vi "Ocean Optics Driver.vi"() -> ()   [LabVIEW 2023]
uses:
  <vilib>/event_ctls.llb/lveventtype.ctl
  <vilib>/Utility/inputDevices.llb/mouseAcquire.vi
  <vilib>/express/express shared/transition.llb/Dynamic To Waveform Array.vi
  <vilib>/express/express signal manip/GetorSetDDTAttributes/Set DDT Attributes/SetT0.vi
  <vilib>/express/express shared/transition.llb/Waveform Array To Dynamic.vi
  <vilib>/express/express signal manip/GetorSetDDTAttributes/Set DDT Attributes/Set DDT Properties.xnode
panel:
  in  "Excitation power:":dbl=84.0 format="%d mW"
  out "Saving Data":bool
  in  "save":bool
  in  "Subtract bckg.":bool
  in  "Background":bool
  in  "length":i32=2 min=0 max=100 step=1
  in  "History mode":bool
  in  "Enable cal":bool
  in  "Calibration consants:":dbl[](array[numeric])=[-1.0164322463e-05, 1.0203031499, -10.120763965] format="%#_6e"
  in  "Raman ref:":dbl=532.0 format="%#_g nm"
  in  "Units":bool=TRUE
  out "Cursor Position:":dbl
  out "XY Graph":cluster{dbl[], "Spectrum Values":dbl[]}[](graph)
  in  "Integration time:":dbl=0.1 min=0.001 max=60.0 step=0.01 format="%#_f s"
  out "Serial Number:":string
  in  "Media Stop Button":bool
  in  "Play":bool
  in  "EXIT":bool
  out "Data":cluster{dbl[], "Spectrum Values":dbl[]}[](array[cluster])
  out "Background":dbl[](array[numeric])
  out "History mode data":cluster{dbl[], "Spectrum Values":dbl[]}[](array[cluster])
  # "2nd:"
  # "1st:"
  # "cm-1"
  # "nm"
  # "0th:"
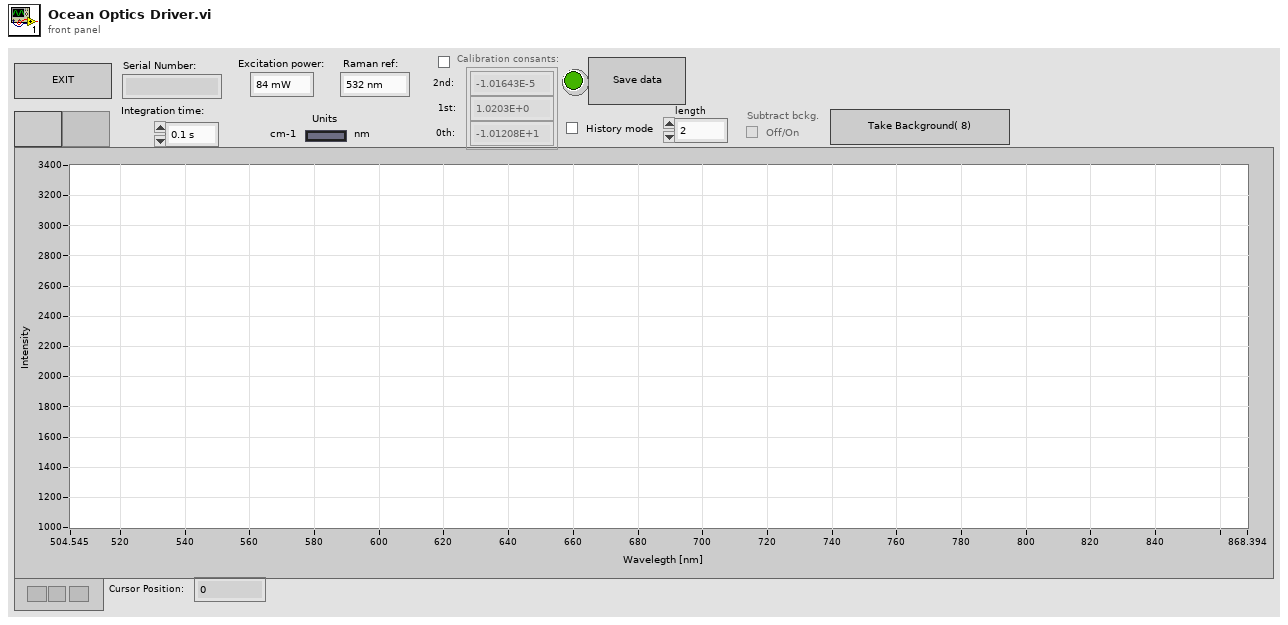
[diagram p1: front panel]
types:
  T1 = enum8{"Enabled", "Disabled", "Disabled and Grayed Out"}
  T2 = typedef "lveventtype.ctl" = enum32{"Null", "Timeout", "Annotation Menu Selection", "Annotation Menu Selection?", "App Instance Close", "App Instance Close?", "Autoscale Range Change", "Bookmark Info Change", "Cell Edit", "Cell Edit?", "Cursor Grab", "Cursor Grab?", "Cursor Menu Selection", "Cursor Menu Selection?", "Cursor Move", "Cursor Release", "Data Change", "Direction Change", "Display State Change", "Drag Ended", "Drag Enter", "Drag Leave", "Drag Over", "Drag Source Update", "Drag Starting", "Drag Starting?", "Drop", "Exec State Change", "Key Down", "Key Down?", "Key Repeat", "Key Repeat?", "Key Up", "Listbox Double Click", "Menu Activation?", "Menu Selection (App)", "Menu Selection? (App)", "Menu Selection (User)", "Mouse Down", "Mouse Down?", "Mouse Enter", "Mouse Leave", "Mouse Move", "Mouse Up", "Mouse Wheel", "NI Security User Change (App)", "Pane Size", "Panel Close", "Panel Close?", "Panel Resize", "Plot Attribute Change", "Scale Range Change", "Shortcut Menu Activation?", "Shortcut Menu Selection (App)", "Shortcut Menu Selection? (App)", "Shortcut Menu Selection (User)", "Tree Double Click", "Tree Drag", "Tree Drag?", "Tree Drop", "Tree Drop?", "Tree Item Close", "Tree Item Close?", "Tree Item Open", "Tree Item Open?", "User Event", "Value Change"}
  T3 = cluster{"Horizontal":i32, "Vertical":i32, "Scrolling":i32}
  T4 = cluster{"button 1":bool, "button 2":bool, "button 3":bool, "button 4":bool}
  T5 = typedef "LVRectTypeDef.ctl" = cluster{"Left":i16, "Top":i16, "Right":i16, "Bottom":i16}
  T6 = cluster{"XScale.Maximum":dbl, "YScale.Maximum":dbl}
  T7 = cluster{"XScale.Minimum":dbl, "YScale.Minimum":dbl}
  T8 = cluster{"event type or object":T2, "event type or object":T2}
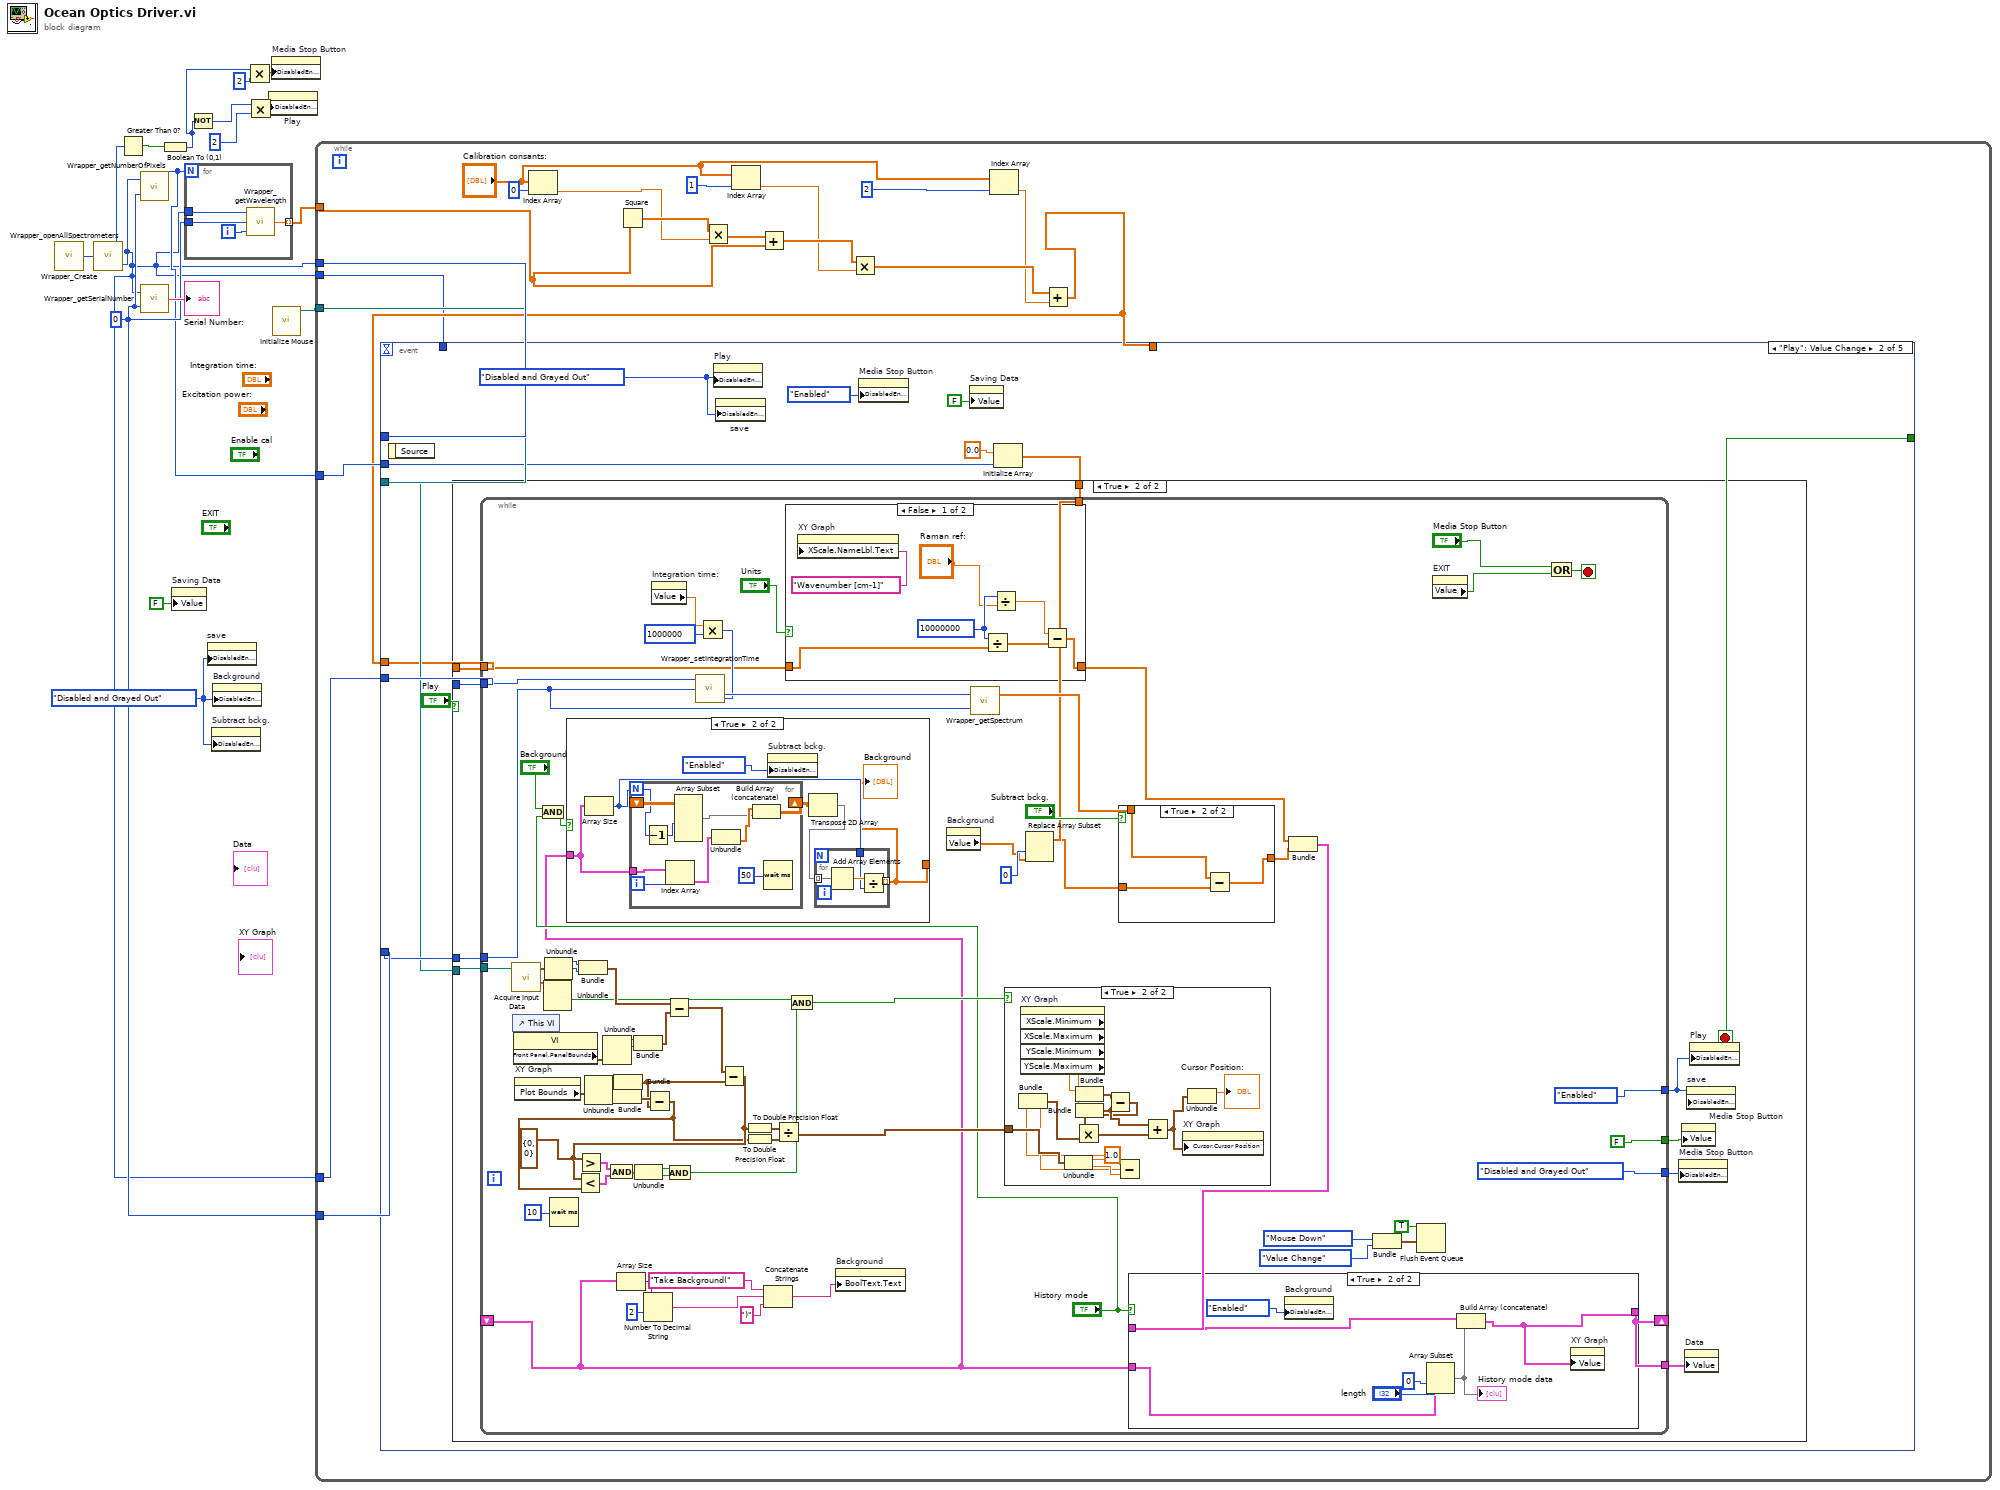
[diagram p0: block diagram]
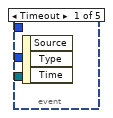
[diagram p2: hidden frame]
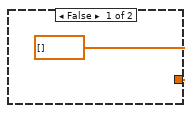
[diagram p5: hidden frame]
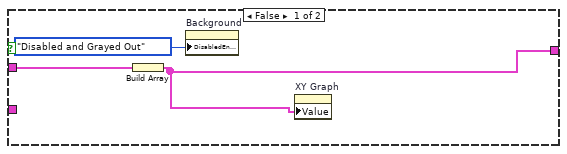
[diagram p6: hidden frame]
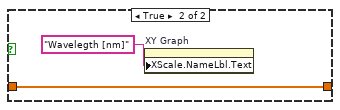
[diagram p7: hidden frame]
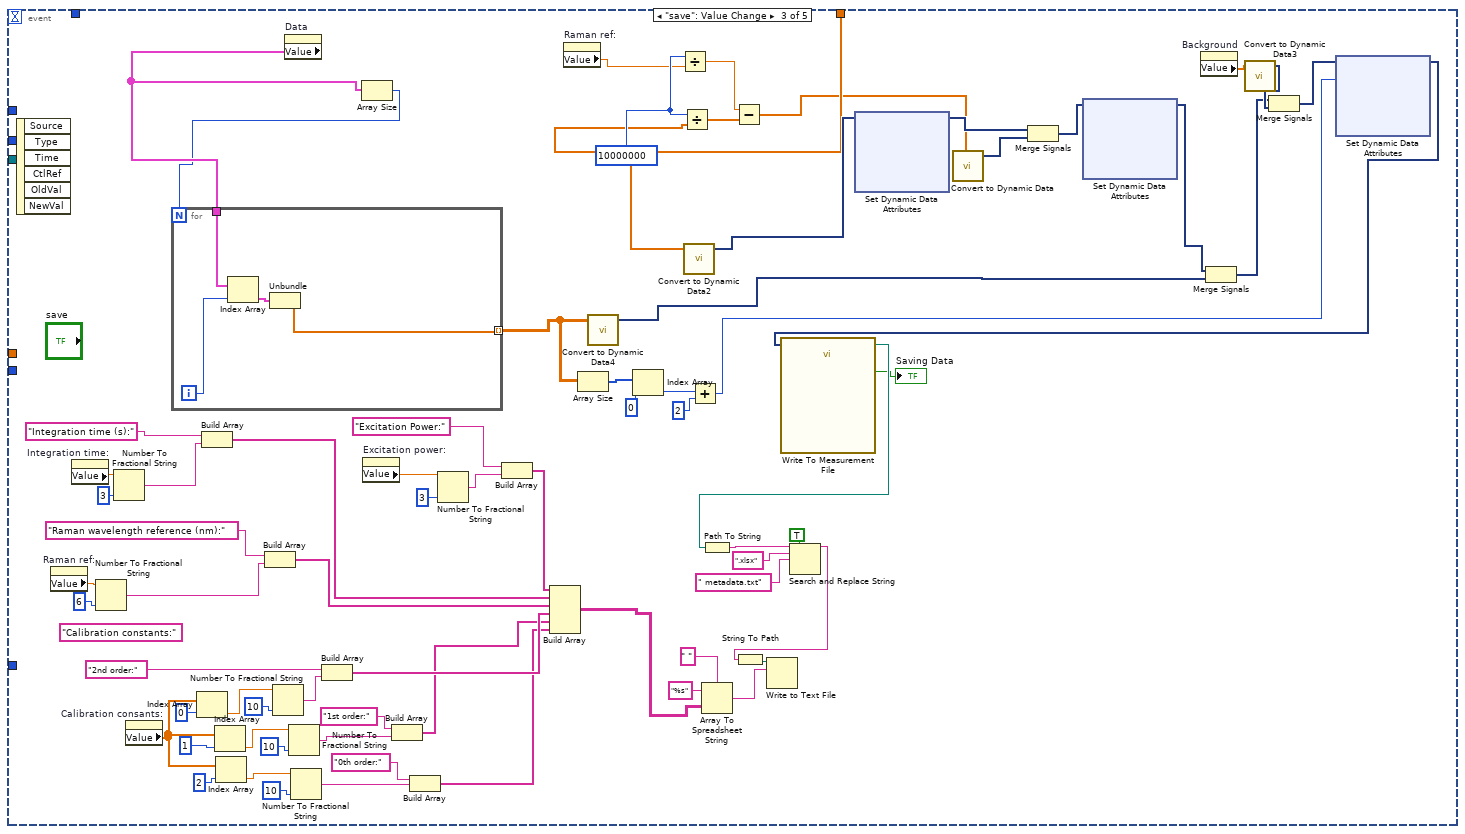
[diagram p9: hidden frame]
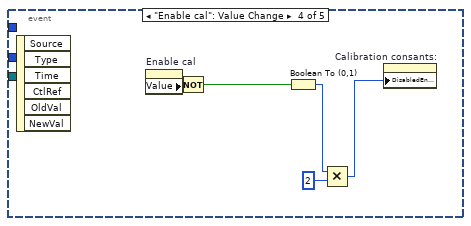
[diagram p10: hidden frame]
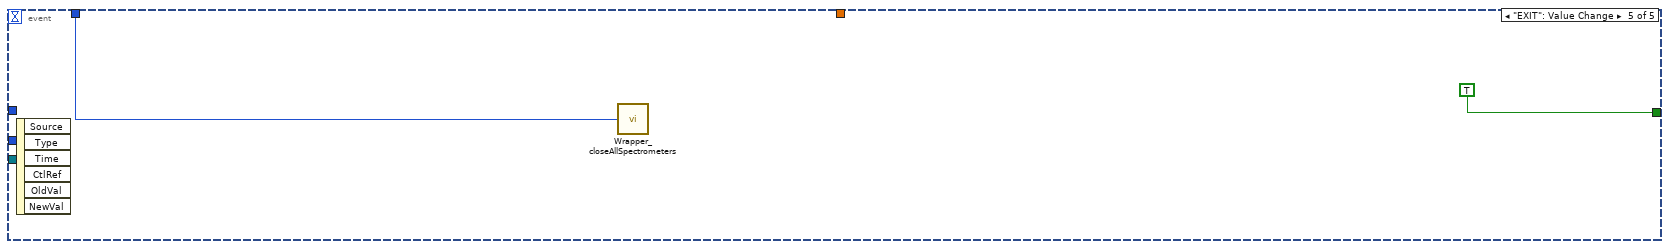
[diagram p11: hidden frame]
diagram:
  w2 = T1."Disabled and Grayed Out" ("Disabled")
  w15 = 0
  n1 = call "Wrapper_Create.vi"() -> ("Wrapper"=w17:u64)
  n2 = call "Wrapper_openAllSpectrometers.vi"("Wrapper In"=w17) -> ("Number of Spectrometers"=w13:i32, "Wrapper Out"=w1:u64)
  n3 = Greater Than 0?(x=w13) -> (x > 0?=w12:bool)
  n4 = call "Wrapper_getNumberOfPixels.vi"("Index"=w15, "Wrapper"=w1) -> ("Number of Pixels"=w4:i32)
  n5 = call "Wrapper_getSerialNumber.vi"("Index"=w15, "Wrapper"=w1) -> ("Serial Number"=→"Serial Number:":string)
  n6 = Boolean To (0,1)(Boolean=w12) -> (0, 1=w6:i16)
  n7 = property on="Saving Data" class="Bool (strict)"("Value"=FALSE ("Saving Data")) -> ()  [unwired: 2 in, 2 out]
  n8 = for {
    N: w4 -> [_]
    tunnel: w1 -> [w21]
    tunnel: w15 -> [w20]
    tunnel: [w18] -> w14 mode=indexing
    i -> [w19]
    n9 = call "Wrapper_getWavelength.vi"("Pixel"=w19, "Spectrometer Index"=w20, "Wrapper"=w21) -> ("Wavelength"=w18:dbl)
  }
  n10 = Not(x=w6) -> (.not. x?=w10:i16)
  n11 = property on="save" class="Bool"("DisabledEnum"=w2) -> ()  [unwired: 2 in, 2 out]
  n12 = property on="Subtract bckg." class="Bool (strict)"("DisabledEnum"=w2) -> ()  [unwired: 2 in, 2 out]
  n13 = property on="Background" class="Bool"("DisabledEnum"=w2) -> ()  [unwired: 2 in, 2 out]
  n14 = Multiply(x=w6, y=2) -> (x*y=w5:i32)
  n15 = Multiply(x=w10, y=2) -> (x*y=w9:i32)
  n16 = property on="Play" class="Bool"("DisabledEnum"=w9) -> ()  [unwired: 2 in, 2 out]
  n17 = property on="Media Stop Button" class="Bool (strict)"("DisabledEnum"=w5) -> ()  [unwired: 2 in, 2 out]
  n18 = call <vilib>:"Initialize Mouse.vi"() -> ("device ID"=w8:refnum<k1>)  [unwired: 10 in, 1 out]
  n19 = while {
    tunnel: w1 -> [w41]
    tunnel: w1 -> [w40]
    tunnel: w15 -> [w39]
    tunnel: w14 -> [w26]
    tunnel: w8 -> [w38]
    tunnel: w4 -> [w25]
    tunnel: w1 -> [w23]
    stop <- w22 stop-if-true
    n20 = Index Array(array="Calibration consants:", index=0) -> (element=w32:dbl)
    n21 = Square(x=w26) -> (x^2=w37:dbl[])
    n22 = Multiply(x=w37, y=w32) -> (x*y=w35:dbl[])
    n23 = Index Array(array="Calibration consants:", index=1) -> (element=w29:dbl)
    n24 = Add(x=w35, y=w26) -> (x+y=w36:dbl[])
    n25 = Multiply(x=w36, y=w29) -> (x*y=w34:dbl[])
    n26 = Index Array(array="Calibration consants:", index=2) -> (element=w28:dbl)
    n27 = Add(x=w34, y=w28) -> (x+y=w24:dbl[])
    n28 = event shown="[1] \"Play\": Value Change" {
      selector: _ -> [_ _ _ _ _]
      dyn-events: _ -> [_ _ _ _ _]
      timeout: _ -> [_ _ _ _ _]
      tunnel: [_ _ _ _ TRUE] -> w22
      tunnel: w41 -> [_ _ _ _ _]
      tunnel: w40 -> [_ w51 _ _ _]
      tunnel: w39 -> [_ w50 _ _ _]
      tunnel: w24 -> [_ w44 _ _ _]
      tunnel: w38 -> [_ w49 _ _ _]
      tunnel: w25 -> [_ w46 _ _ _]
      tunnel: w24 -> [_ _ w236 _ _]
      tunnel: w23 -> [_ _ _ _ w315]
      event Timeout {
        n29 = event-data() -> ()  [unwired: 1 in, 3 out]
      }
      event "Play": Value Change {
        w42 = T1."Disabled and Grayed Out" ("Disabled")
        n30 = event-data() -> ()  [unwired: 1 in, 1 out]
        n31 = property on="Play" class="Bool"("DisabledEnum"=w42) -> ()  [unwired: 2 in, 2 out]
        n32 = property on="save" class="Bool"("DisabledEnum"=w42) -> ()  [unwired: 2 in, 2 out]
        n33 = property on="Media Stop Button" class="Bool (strict)"("DisabledEnum"=T1."Enabled" ("Disabled")) -> ()  [unwired: 2 in, 2 out]
        n34 = property on="Saving Data" class="Bool (strict)"("Value"=FALSE ("Saving Data")) -> ()  [unwired: 2 in, 2 out]
        n35 = Initialize Array(0.0 ("element"), w46) -> (w45:dbl[])
        n36 = case shown="True" "Play" {
          tunnel: w51 -> [_ w61]
          tunnel: w50 -> [_ w60]
          tunnel: w44 -> [_ w59]
          tunnel: w49 -> [_ w58]
          tunnel: w45 -> [_ w55]
          frame False {
          }
          frame True {
            n37 = while {
              tunnel: w61 -> [w98]
              tunnel: w60 -> [w96]
              tunnel: w59 -> [w87]
              tunnel: w58 -> [w131]
              tunnel: [T1."Disabled and Grayed Out" ("Disabled")] -> w57
              tunnel: [FALSE ("Media Stop Button")] -> w56
              shift-right: [w72] -> _
              shift-left: _ -> [w63]
              tunnel: w55 -> [w78]
              tunnel: [T1."Enabled" ("Disabled")] -> w53
              tunnel: [w72] -> w54
              stop <- w133 stop-if-true
              n38 = call-poly <vilib>:"Acquire Input Data.vi"("device ID"=w131) -> ("axis info"=w127:T3, "button info"=w130:T4)  [unwired: 15 in, 2 out]
              n39 = control-ref of="This VI"() -> (w118:refnum<vi>)
              n40 = property class="VI"(reference=w118) -> ("Front Panel.PanelBounds"=w119:T5)  [unwired: 1 in, 2 out]
              n41 = property on="XY Graph" class="XYGraph (strict)"() -> ("Plot Bounds"=w123:T5)  [unwired: 2 in, 2 out]
              n42 = And(x="Background", y="History mode") -> (x .and. y?=w83:bool)
              n43 = Unbundle(w130) -> ("button 1"=w113:bool)  [unwired: 3 out]
              n44 = Unbundle(w127) -> ("Horizontal"=w128:i32, "Vertical"=w129:i32)  [unwired: 1 out]
              n45 = Wait (ms)(milliseconds to wait=u32 10) -> ()  [unwired: 1 out]
              n46 = case shown="True" w83 {
                tunnel: w63 -> [_ w144]
                tunnel: [dbl[] [] w140] -> _
                frame False {
                }
                frame True {
                  n47 = Array Size(array=w144) -> (size(s)=w141:i32)
                  n48 = for {
                    N: w141 -> [w150]
                    tunnel: w144 -> [w156]
                    shift-right: [w154] -> w143
                    shift-left: _ -> [w152]
                    i -> [w155]
                    n49 = Decrement(x=w150) -> (x-1=w149:i32)
                    n50 = Index Array(array=w156, index=w155) -> (element=w158:cluster{dbl[], "Spectrum Values":dbl[]})
                    n51 = Array Subset(array=w152, length (row)=w149) -> (w151:dbl[][])  [unwired: 3 in]
                    n52 = Unbundle(w158) -> ("Spectrum Values"=w153:dbl[])  [unwired: 1 out]
                    n53 = Build Array (concatenate)(w153, w151) -> (w154:dbl[][])
                    n54 = Wait (ms)(milliseconds to wait=u32 50) -> ()  [unwired: 1 out]
                  }
                  n55 = property on="Subtract bckg." class="Bool (strict)"("DisabledEnum"=T1."Enabled" ("Disabled")) -> ()  [unwired: 2 in, 2 out]
                  n56 = Transpose 2D Array(2D array=w143) -> (transposed array=w142:dbl[][])
                  n57 = for {
                    tunnel: w142 -> [w148] mode=indexing
                    tunnel: [w145] -> w140 mode=indexing
                    tunnel: w141 -> [w146]
                    n58 = Add Array Elements(numeric array=w148) -> (sum=w147:dbl)
                    n59 = Divide(x=w147, y=w146) -> (x/y=w145:dbl)
                  }
                  "Background" <- w140
                }
              }
              n60 = Bundle("Horizontal"=w128, "Vertical"=w129) -> (w126:cluster{"Horizontal":i32, "Vertical":i32})  [unwired: 1 in]
              n61 = Unbundle(w123) -> ("Left"=w124:i16, "Top"=w125:i16, "Right"=w108:i16, "Bottom"=w107:i16)
              n62 = Unbundle(w119) -> ("Left"=w120:i16, "Top"=w122:i16)  [unwired: 2 out]
              n63 = Bundle("Right"=w108, "Bottom"=w107) -> (w105:cluster{"Right":i16, "Bottom":i16})  [unwired: 1 in]
              n64 = Bundle("Left"=w124, "Top"=w125) -> (w104:cluster{"Left":i16, "Top":i16})  [unwired: 1 in]
              n65 = Array Size(array=w63) -> (size(s)=w67:i32)
              n66 = Bundle("Left"=w120, "Top"=w122) -> (w121:cluster{"Left":i16, "Top":i16})  [unwired: 1 in]
              n67 = Number To Decimal String(number=w67, width (-)=i16 2) -> (decimal integer string=w68:string)
              n68 = Subtract(x=w105, y=w104) -> (x-y=w102:cluster{i16, i16})
              n69 = property on="Integration time:" class="DigNum (strict)"() -> ("Value"=w94:dbl)  [unwired: 2 in, 2 out]
              n70 = Subtract(x=w126, y=w121) -> (x-y=w106:cluster{i32, i32})
              n71 = Multiply(x=w94, y=1000000) -> (x*y=w93:i32)
              n72 = call "Wrapper_setIntegrationTime.vi"("Integration Time"=w93, "Index"=w96, "Wrapper In"=w98) -> ("Wrapper Out"=w97:u64)
              n73 = Subtract(x=w106, y=w104) -> (x-y=w103:cluster{i32, i32})
              n74 = Less?(x=w103, y=w102) -> (x < y?=w116:cluster{bool, bool})
              n75 = Greater?(x=w103, y=cluster{i32, i32} {0, 0}) -> (0:w115:cluster{bool, bool})
              n76 = And(x=w115, y=w116) -> (x .and. y?=w114:cluster{bool, bool})
              n77 = Unbundle(w114) -> (w111:bool, w110:bool)
              n78 = And(x=w111, y=w110) -> (x .and. y?=w109:bool)
              n79 = To Double Precision Float(number=w103) -> (double precision float=w100:cluster{dbl, dbl})
              n80 = To Double Precision Float(number=w102) -> (double precision float=w101:cluster{dbl, dbl})
              n81 = Concatenate Strings("Take Background(" ("string"), w68, ")" ("string")) -> (w69:string)
              n82 = Divide(x=w100, y=w101) -> (x/y=w99:cluster{dbl, dbl})
              n83 = case shown="False" "Units" {
                tunnel: [w170 w176] -> w71
                tunnel: w87 -> [w172 w176]
                frame False {
                  w174 = 10000000 ("x")
                  n84 = property on="XY Graph" class="XYGraph (strict)"("XScale.NameLbl.Text"="Wavenumber [cm-1]" ("X Scale.Name Label.Text")) -> ()  [unwired: 2 in, 2 out]
                  n85 = Divide(x=w174, y=w172) -> (x/y=w171:dbl[])
                  n86 = Divide(x=w174, y="Raman ref:") -> (x/y=w173:dbl)
                  n87 = Subtract(x=w173, y=w171) -> (x-y=w170:dbl[])
                }
                frame True {
                  n88 = property on="XY Graph" class="XYGraph (strict)"("XScale.NameLbl.Text"="Wavelegth [nm]" ("X Scale.Name Label.Text")) -> ()  [unwired: 2 in, 2 out]
                }
              }
              n89 = And(x=w113, y=w109) -> (x .and. y?=w112:bool)
              n90 = property on="Background" class="Bool"("BoolText.Text"=w69) -> ()  [unwired: 2 in, 2 out]
              n91 = property on="Background" class="Arr (strict)"() -> ("Value"=w75:dbl[])  [unwired: 2 in, 2 out]
              n92 = call "Wrapper_getSpectrum.vi"("Index"=w96, "Wrapper"=w97) -> ("Spectrum Values"=w79:dbl[])  [unwired: 1 out]
              n93 = case shown="True" w112 {
                tunnel: w99 -> [_ w186]
                frame False {
                }
                frame True {
                  n94 = property on="XY Graph" class="XYGraph (strict)"() -> ("XScale.Minimum"=w191:dbl, "XScale.Maximum"=w193:dbl, "YScale.Minimum"=w190:dbl, "YScale.Maximum"=w192:dbl)  [unwired: 2 in, 2 out]
                  n95 = Unbundle(w186) -> (w182:dbl, w184:dbl)
                  n96 = Bundle("XScale.Maximum"=w193, "YScale.Maximum"=w192) -> (w188:T6)  [unwired: 1 in]
                  n97 = Bundle("XScale.Minimum"=w191, "YScale.Minimum"=w190) -> (w189:T7)  [unwired: 1 in]
                  n98 = Subtract(x=w188, y=w189) -> (x-y=w181:cluster{dbl, dbl})
                  n99 = Subtract(x=1.0, y=w184) -> (x-y=w183:dbl)
                  n100 = Bundle(w182, w183) -> (w180:cluster{dbl, dbl})  [unwired: 1 in]
                  n101 = Multiply(x=w181, y=w180) -> (x*y=w187:cluster{dbl, dbl})
                  n102 = Add(x=w189, y=w187) -> (x+y=w179:cluster{dbl, dbl})
                  n103 = property on="XY Graph" class="XYGraph (strict)"("Cursor.Cursor Position"=w179) -> ()  [unwired: 2 in, 2 out]
                  n104 = Unbundle(w179) -> (→"Cursor Position:":dbl)  [unwired: 1 out]
                }
              }
              n105 = Replace Array Subset(array=w78, new element=w75, index=0) -> (w77:dbl[])
              n106 = case shown="True" "Subtract bckg." {
                tunnel: [w134 w136] -> w80
                tunnel: w79 -> [w134 w137]
                tunnel: w77 -> [_ w135]
                frame False {
                }
                frame True {
                  n107 = Subtract(x=w137, y=w135) -> (x-y=w136:dbl[])
                }
              }
              n108 = Bundle(w71, "Spectrum Values"=w80) -> (w82:cluster{dbl[], "Spectrum Values":dbl[]})  [unwired: 1 in]
              n109 = case shown="True" "History mode" {
                tunnel: [w160 w165] -> w72
                tunnel: w63 -> [_ w162]
                tunnel: w82 -> [w161 w163]
                frame False {
                  n110 = Build Array(w161) -> (w160:cluster{dbl[], "Spectrum Values":dbl[]}[])
                  n111 = property on="Background" class="Bool"("DisabledEnum"=T1."Disabled and Grayed Out" ("Disabled")) -> ()  [unwired: 2 in, 2 out]
                  n112 = property on="XY Graph" class="XYGraph (strict)"("Value"=w160) -> ()  [unwired: 2 in, 2 out]
                }
                frame True {
                  n113 = property on="Background" class="Bool"("DisabledEnum"=T1."Enabled" ("Disabled")) -> ()  [unwired: 2 in, 2 out]
                  n114 = Array Subset(array=w162, index=0, length="length") -> (w166:cluster{dbl[], "Spectrum Values":dbl[]}[])
                  "History mode data" <- w166
                  n115 = Build Array (concatenate)(w163, w166) -> (w165:cluster{dbl[], "Spectrum Values":dbl[]}[])
                  n116 = property on="XY Graph" class="XYGraph (strict)"("Value"=w165) -> ()  [unwired: 2 in, 2 out]
                }
              }
              n117 = Bundle("event type or object"=lveventtype."Mouse Down", "event type or object"=lveventtype."Value Change") -> (w90:T8)  [unwired: 1 in]
              n118 = Flush Event Queue(1:TRUE ("include static events? (T)"), 2:w90) -> ()  [unwired: 4 in, 3 out]
              n119 = property on="EXIT" class="Bool (strict)"() -> ("Value"=w132:bool)  [unwired: 2 in, 2 out]
              n120 = Or(x="Media Stop Button", y=w132) -> (x .or. y?=w133:bool)
            }
            n121 = property on="Media Stop Button" class="Bool (strict)"("DisabledEnum"=w57) -> ()  [unwired: 2 in, 2 out]
            n122 = property on="Media Stop Button" class="Bool (strict)"("Value"=w56) -> ()  [unwired: 2 in, 2 out]
            n123 = property on="Data" class="Arr (strict)"("Value"=w54) -> ()  [unwired: 2 in, 2 out]
            n124 = property on="save" class="Bool"("DisabledEnum"=w53) -> ()  [unwired: 2 in, 2 out]
            n125 = property on="Play" class="Bool"("DisabledEnum"=w53) -> ()  [unwired: 2 in, 2 out]
          }
        }
      }
      event "save": Value Change {
        w241 = 10000000 ("x")
        (unwired) "Calibration constants:" ("element")
        n126 = event-data() -> ()  [unwired: 1 in, 6 out]
        n127 = property on="Raman ref:" class="DigNum (strict)"() -> ("Value"=w252:dbl)  [unwired: 2 in, 2 out]
        n128 = property on="Integration time:" class="DigNum (strict)"() -> ("Value"=w254:dbl)  [unwired: 2 in, 2 out]
        n129 = Number To Fractional String(number=w252, precision (6)=i16 6 ("width (-)")) -> (F-format string=w218:string)  [unwired: 2 in]
        n130 = Number To Fractional String(number=w254, precision (6)=i16 3 ("width (-)")) -> (F-format string=w220:string)  [unwired: 2 in]
        n131 = property on="Calibration consants:" class="Arr (strict)"() -> ("Value"=w248:dbl[])  [unwired: 2 in, 2 out]
        n132 = Index Array(array=w248, index=0) -> (element=w244:dbl)
        n133 = Build Array("Integration time (s):", w220) -> (w211:string[])
        n134 = Index Array(array=w248, index=1) -> (element=w243:dbl)
        n135 = Index Array(array=w248, index=2) -> (element=w242:dbl)
        n136 = Build Array("Raman wavelength reference (nm):" ("element"), w218) -> (w210:string[])
        n137 = Number To Fractional String(number=w244, precision (6)=i16 10 ("width (-)")) -> (F-format string=w216:string)  [unwired: 2 in]
        n138 = property on="Data" class="Arr (strict)"() -> ("Value"=w264:cluster{dbl[], "Spectrum Values":dbl[]}[])  [unwired: 2 in, 2 out]
        n139 = Number To Fractional String(number=w243, precision (6)=i16 10 ("width (-)")) -> (F-format string=w215:string)  [unwired: 2 in]
        n140 = Number To Fractional String(number=w242, precision (6)=i16 10 ("width (-)")) -> (F-format string=w213:string)  [unwired: 2 in]
        n141 = Build Array("2nd order:" ("element"), w216) -> (w209:string[])
        n142 = Array Size(array=w264) -> (size(s)=w263:i32)
        n143 = for {
          N: w263 -> [_]
          tunnel: w264 -> [w309]
          tunnel: [w306] -> w203 mode=indexing
          i -> [w308]
          n144 = Index Array(array=w309, index=w308) -> (element=w307:cluster{dbl[], "Spectrum Values":dbl[]})
          n145 = Unbundle(w307) -> ("Spectrum Values"=w306:dbl[])  [unwired: 1 out]
        }
        n146 = property on="Excitation power:" class="DigNum (strict)"() -> ("Value"=w228:dbl)  [unwired: 2 in, 2 out]
        n147 = Build Array("1st order:" ("element"), w215) -> (w208:string[])
        n148 = Build Array("0th order:" ("element"), w213) -> (w207:string[])
        n149 = Number To Fractional String(number=w228, precision (6)=i16 3) -> (F-format string=w223:string)  [unwired: 2 in]
        n150 = Build Array("Excitation Power:" ("element"), w223) -> (w222:string[])
        n151 = Build Array(w222, w211, w210, w209, w208, w207) -> (w205:string[][])
        n152 = property on="Raman ref:" class="DigNum (strict)"() -> ("Value"=w238:dbl)  [unwired: 2 in, 2 out]
        n153 = Array Size(array=w203) -> (size(s)=w202:i32[])
        n154 = call "Convert to Dynamic Data4"("2D Array"=w203) -> ("Dynamic Data Type"=w229:dynamicdata)  [unwired: 3 in]
        n155 = Index Array(array=w202, index=0) -> (element=w200:i32)
        n156 = Divide(x=w241, y=w238) -> (x/y=w240:dbl)
        n157 = Divide(x=w241, y=w236) -> (x/y=w239:dbl[])
        n158 = call "Convert to Dynamic Data2"("Array"=w236) -> ("Dynamic Data Type"=w237:dynamicdata)  [unwired: 3 in]
        n159 = Add(x=w200, y=2) -> (x+y=w198:i32)
        n160 = Array To Spreadsheet String(delimiter (Tab)=" ", array=w205, 3:"%s" ("format string")) -> (spreadsheet string=w226:string)
        n161 = Subtract(x=w240, y=w239) -> (x-y=w233:dbl[])
        n162 = xnode "Set Dynamic Data Attributes"("Signals In"=w237) -> ("Signals Out"=w234:dynamicdata)  [unwired: 3 in, 1 out]
        n163 = call "Convert to Dynamic Data"("Array"=w233) -> ("Dynamic Data Type"=w232:dynamicdata)  [unwired: 3 in]
        n164 = Merge Signals(w234, w232) -> (w231:dynamicdata)
        n165 = xnode "Set Dynamic Data Attributes"("Signals In"=w231) -> ("Signals Out"=w230:dynamicdata)  [unwired: 3 in, 1 out]
        n166 = property on="Background" class="Arr (strict)"() -> ("Value"=w204:dbl[])  [unwired: 2 in, 2 out]
        n167 = Merge Signals(w230, w229) -> (w194:dynamicdata)
        n168 = call "Convert to Dynamic Data3"("Array"=w204) -> ("Dynamic Data Type"=w195:dynamicdata)  [unwired: 3 in]
        n169 = Merge Signals(w194, w195) -> (w197:dynamicdata)
        n170 = xnode "Set Dynamic Data Attributes"("Signals In"=w197, "Signal Index"=w198) -> ("Signals Out"=w196:dynamicdata)  [unwired: 2 in, 1 out]
        n171 = call "Write To Measurement File"("Signals"=w196) -> ("Filename Out"=w258:path, "Saving Data"=→"Saving Data":bool)  [unwired: 16 in, 1 out]
        n172 = Path To String(path=w258) -> (string=w262:string)
        n173 = Search and Replace String(replace all?=TRUE ("replace all? (F)"), input string=w262, search string=".xlsx", replace string=" metadata.txt" ("replace string (\"\")")) -> (result string=w257:string)  [unwired: 4 in, 3 out]
        n174 = String To Path(string=w257) -> (path=w256:path)
        n175 = Write to Text File(file (use dialog)=w256, text=w226) -> ()  [unwired: 2 in, 3 out]
      }
      event "Enable cal": Value Change {
        n176 = event-data() -> ()  [unwired: 1 in, 6 out]
        n177 = property on="Enable cal" class="Bool (strict)"() -> ("Value"=w311:bool)  [unwired: 2 in, 2 out]
        n178 = Not(x=w311) -> (.not. x?=w310:bool)
        n179 = Boolean To (0,1)(Boolean=w310) -> (0, 1=w314:i16)
        n180 = Multiply(x=w314, y=i16 2) -> (x*y=w312:i16)
        n181 = property on="Calibration consants:" class="Arr (strict)"("DisabledEnum"=w312) -> ()  [unwired: 2 in, 2 out]
      }
      event "EXIT": Value Change {
        n182 = event-data() -> ()  [unwired: 1 in, 6 out]
        n183 = call "Wrapper_closeAllSpectrometers.vi"("Wrapper In"=w315) -> ()  [unwired: 1 out]
      }
    }
  }
